vi "Create Custom Device.vi"(0 "Name":string, 5 "AIT 664 Settings":T1, 11 "error in (no error)":errorcluster) -> (4 "Custom Device reference":refnum<k24>, 15 "error out":errorcluster)   [LabVIEW 2015]
uses:
  NationalInstruments.VeriStand.SystemDefinitionAPI
  Controls/AIT 664 Settings.ctl
  Controls and Global/Global.vi
  AIT 664 Custom Device.lvlib
  <vilib>/NI Veristand/Custom Device API/Custom Device API.lvlib
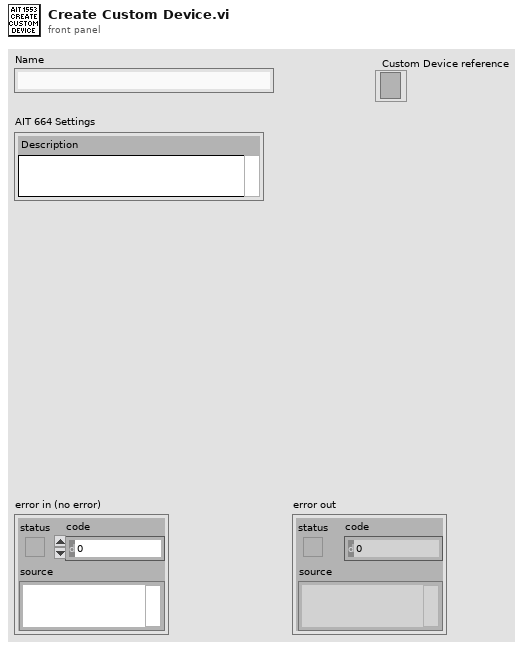
[diagram p1: front panel]
types:
  T1 = typedef "AIT 664 Settings.ctl" = cluster{"Description":string}
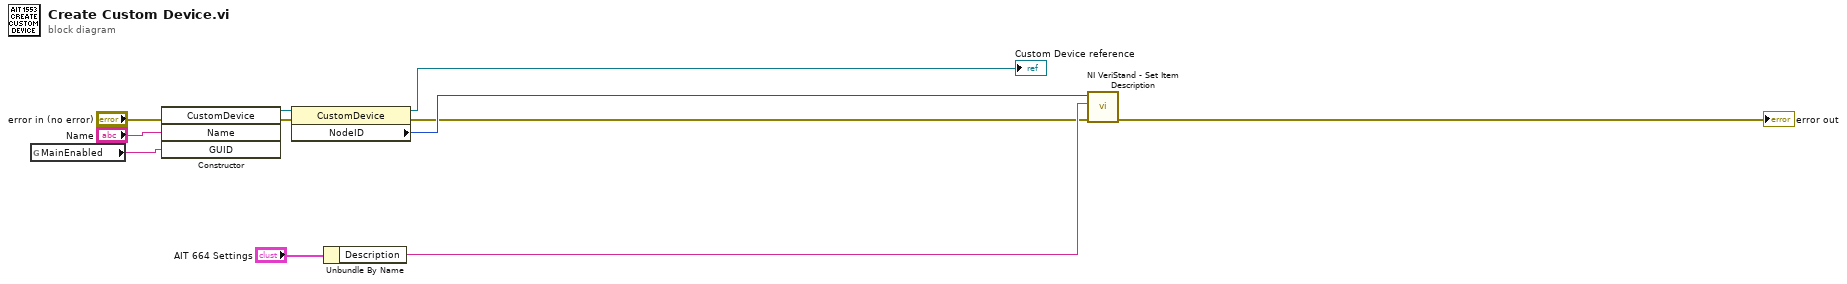
[diagram p0: block diagram]
diagram:
  n1 = global read "Global.vi" "MainEnabled"() -> (w7:string)
  n2 = constructor class="CustomDevice"(error in="error in (no error)", "Name"="Name", "GUID"=w7) -> (reference out=w10:refnum<k24>, error out=w11:errorcluster)  [unwired: 2 in, 3 out]
  n3 = property class="CustomDevice"(reference=w10, error in=w11) -> (reference out=→"Custom Device reference":refnum<k24>, error out=w1:errorcluster, "NodeID"=w2:u64)
  n4 = Unbundle By Name("AIT 664 Settings") -> ("Description"=w5:string)
  n5 = call <vilib>:"NI VeriStand - Set Item Description.vi"("error in (no error)"=w1, "Description"=w5, "Item Ref in"=w2) -> ("error out"=→"error out":errorcluster)  [unwired: 8 out]
